vi "AIM 664 test Add-Find-Remove Custom Device.vi"(8 "error in":errorcluster, 11 "TestCase in":refnum<class "AIM 664 Scripting.lvclass">) -> (0 "error out":errorcluster, 3 "TestCase out":refnum<class "AIM 664 Scripting.lvclass">)   [LabVIEW 2020, in "AIM 664 Scripting.lvclass"]
uses:
  AIM 664 Scripting.lvclass
  C:/Program Files (x86)/National Instruments/LabVIEW 2020/vi.lib/NI/VeriStand Custom Device Testing Tools/VeriStandScriptingTestCase/VeriStandScriptingTestCase.lvclass
  <vilib>/NI/VeriStand Custom Device Testing Tools/VeriStandScriptingTestCase/VeriStandScriptingTestCase.lvclass/VeriStandScriptingTestCase.ctl
  <vilib>/NI/VeriStand Custom Device Testing Tools/VeriStandScriptingTestCase/Read Target.vi
  NationalInstruments.VeriStand.SystemDefinitionAPI
  <vilib>/addons/_JKI Toolkits/VI Tester/TestCase.llb/TestCase.lvclass
  Scripting/AIM ARINC 664 Scripting.lvlib
  C:/Program Files (x86)/National Instruments/LabVIEW 2020/vi.lib/addons/_JKI Toolkits/VI Tester/TestCase.llb/TestCase.lvclass
  C:/repos/niveristand-aim-arinc664-custom-device/Source/Custom Device Support/Tests/Unit/Scripting/AIM 664 Scripting.lvclass
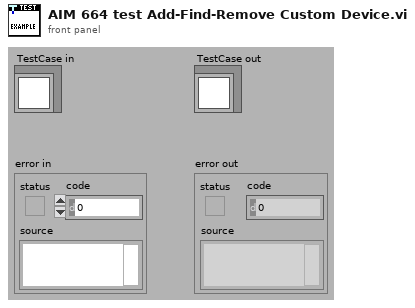
[diagram p1: front panel]
types:
  T1 = typedef "Custom Device API.lvlib/Custom Device Item Ref.ctl" = u64
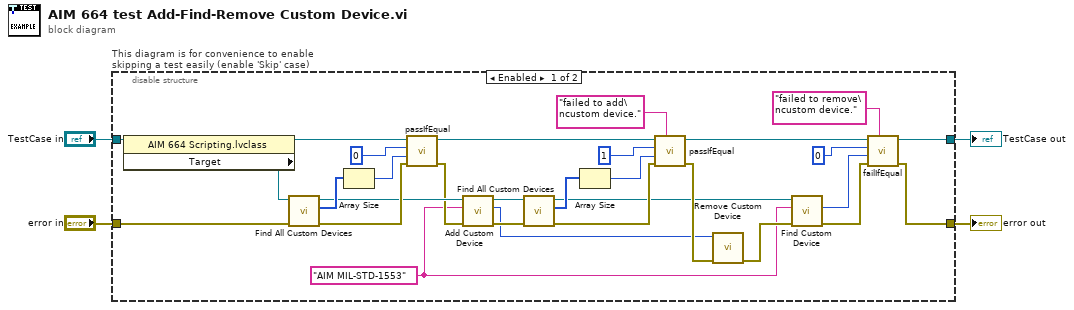
[diagram p0: block diagram]
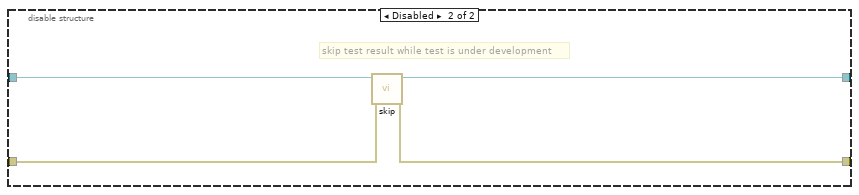
[diagram p2: hidden frame]
diagram:
  n1 = disable-structure "This diagram is for convenience to enable skipping a test easily (enable 'Skip' case)" shown="Enabled" {
    disable-tunnel: "TestCase in" -> [w27 w38]
    disable-tunnel: [w28 w36] -> w1
    disable-tunnel: [w29 w37] -> w3
    disable-tunnel: "error in" -> [w24 w35]
    frame Enabled {
      w10 = "AIM MIL-STD-1553" ("name")
      n2 = property class="AIM 664 Scripting.lvclass"(reference=w27) -> (reference out=w26:refnum<class "AIM 664 Scripting.lvclass">, "Target"=w21:refnum<k24>)  [unwired: 1 in, 1 out]
      n3 = call "Find All Custom Devices.vi"("error in"=w24, "target in"=w21) -> ("error out"=w23:errorcluster, "custom devices"=w22:u64[], "target out"=w20:refnum<k24>)  [unwired: 7 in]
      n4 = Array Size(array=w22) -> (size(s)=w34:i32)
      n5 = call-dynamic "passIfEqual.vi"("error in (no error)"=w23, "y"=w34, "x"=0 ("size(s)"), "TestCase in"=w26) -> ("error out"=w19:errorcluster, "TestCase out"=w25:refnum<class "AIM 664 Scripting.lvclass">)  [unwired: 6 in]
      n6 = call "Add Custom Device.vi"("error in"=w19, "name"=w10, "target in"=w20) -> ("error out"=w18:errorcluster, "custom device"=w13:T1, "target out"=w16:refnum<k24>)  [unwired: 6 in]
      n7 = call "Find All Custom Devices.vi"("error in"=w18, "target in"=w16) -> ("error out"=w17:errorcluster, "custom devices"=w15:u64[], "target out"=w9:refnum<k24>)  [unwired: 7 in]
      n8 = Array Size(array=w15) -> (size(s)=w31:i32)
      n9 = call-dynamic "passIfEqual.vi"("custom report message (\"\")"="failed to add\ncustom device." ("custom report message (\"\")"), "error in (no error)"=w17, "y"=w31, "x"=1 ("size(s)"), "TestCase in"=w25) -> ("error out"=w14:errorcluster, "TestCase out"=w30:refnum<class "AIM 664 Scripting.lvclass">)  [unwired: 5 in]
      n10 = call "Remove Custom Device.vi"("error in"=w14, "custom device"=w13) -> ("error out"=w11:errorcluster)  [unwired: 9 in]
      n11 = call "Find Custom Device.vi"("error in"=w11, "name"=w10, "target in"=w9) -> ("error out"=w12:errorcluster, "custom device"=w8:u64)  [unwired: 6 in, 1 out]
      n12 = call-dynamic "failIfEqual.vi"("custom report message (\"\")"="failed to remove\ncustom device." ("custom report message (\"\")"), "error in (no error)"=w12, "y"=w8, "x"=0 ("size(s)"), "TestCase in"=w30) -> ("error out"=w29:errorcluster, "TestCase out"=w28:refnum<class "AIM 664 Scripting.lvclass">)  [unwired: 5 in]
    }
    frame Disabled {
      # "skip test result while test is under development"
      n13 = call <vilib>:"skip.vi"("error in (no error)"=w35, "TestCase in"=w38) -> ("error out"=w37:errorcluster, "TestCase out"=w36:refnum<class "AIM 664 Scripting.lvclass">)  [unwired: 8 in]
    }
  }
  "error out" <- w3
  "TestCase out" <- w1
